vi "Set Password.vi"(8 "error in (no error)":errorcluster, 9 "New password":string, 10 "ProjectItem Refnum":refnum<vi>, 11 "DLL in":refnum<class "NI_AB_API_DLL.lvclass">) -> (0 "error out":errorcluster, 3 "DLL out":refnum<class "NI_AB_API_DLL.lvclass">)   [LabVIEW 2020, in "NI_AB_API_DLL.lvclass"]
uses:
  <vilib>/AppBuilder/AB_API/DLL/NI_AB_API_DLL.lvclass
  <vilib>/AppBuilder/AB_API/Application/NI_AB_API_Application.lvclass
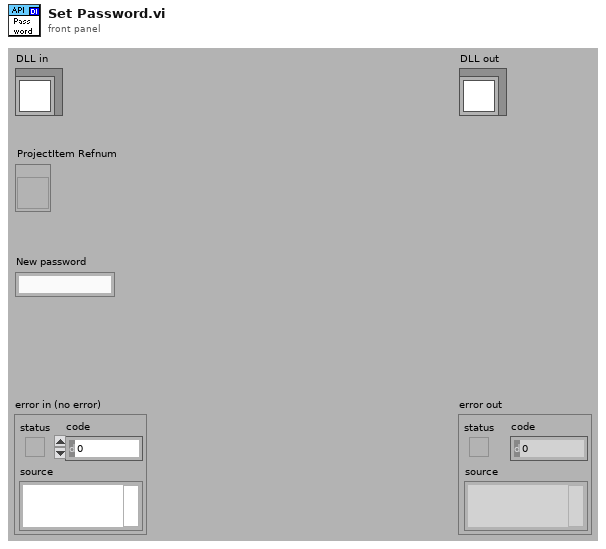
[diagram p1: front panel]
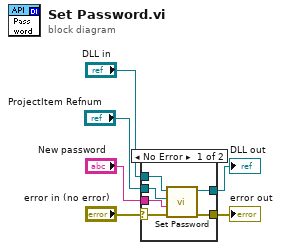
[diagram p0: block diagram]
diagram:
  n1 = case shown="No Error" "error in (no error)" {
    selector: "error in (no error)" -> [w9 w14]
    tunnel: [w10 w14] -> w5
    tunnel: [w11 w13] -> w3
    tunnel: "DLL in" -> [w12 w13]
    tunnel: "ProjectItem Refnum" -> [w7 _]
    tunnel: "New password" -> [w8 _]
    frame No Error {
      n2 = call-parent "Set Password.vi"("error in (no error)"=w9, "New password"=w8, "ProjectItem Refnum"=w7, "Build in"=w12) -> ("error out"=w10:errorcluster, "Build out"=w11:refnum<class "NI_AB_API_DLL.lvclass">)  [unwired: 6 in]
    }
    frame Error {
    }
  }
  "error out" <- w5
  "DLL out" <- w3
